vi "CleanUp.vi"(5 "Error In":errorcluster) -> (19 "Error Out":errorcluster)   [LabVIEW 2020, in "SingletonTemplate.lvclass"]
uses:
  SingletonTemplate.lvclass
  SingletonTemplate.lvclass/SingletonTemplate.ctl
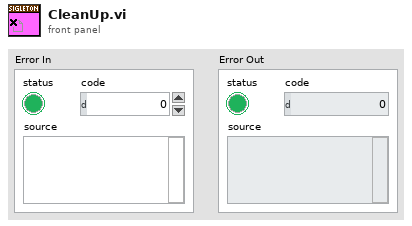
[diagram p1: front panel]
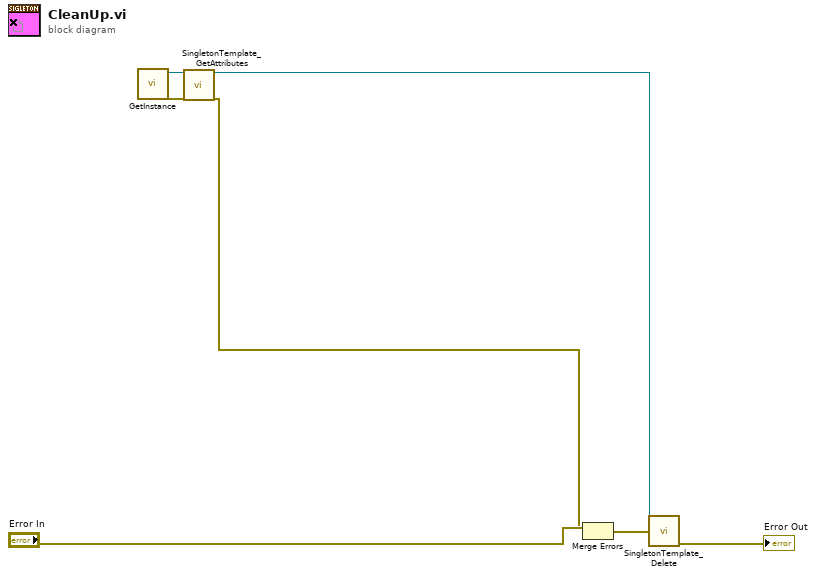
[diagram p0: block diagram]
diagram:
  n1 = call "GetInstance.vi"() -> ("reference out"=w2:refnum<class "SingletonTemplate.lvclass">, "error out"=w1:errorcluster)  [unwired: 18 in]
  n2 = call "SingletonTemplate_GetAttributes.vi"("reference in"=w2, "error in (no error)"=w1) -> ("reference out"=w5:refnum<class "SingletonTemplate.lvclass">, "error out"=w3:errorcluster)  [unwired: 14 in, 2 out]
  n3 = Merge Errors("Error In", w3) -> (w4:errorcluster)
  n4 = call "SingletonTemplate_Delete.vi"("reference in"=w5, "error in (no error)"=w4) -> ("error out"=→"Error Out":errorcluster)  [unwired: 15 in, 2 out]
